vi "Open Selected VI Location.vi"(6 "Variant in":variant, 7 "Shift Pressed?":bool, 8 "error in (no error)":errorcluster, 10 "QD Combo Box Ref":refnum<vi>, 11 "QD Launch VI Ref":refnum<vi>) -> (0 "error out":errorcluster, 4 "Variant out":variant)   [LabVIEW 2017, in "Smart Open VI Location.lvlib"]
doc: "Open Selected VI's Location in Explorer Window."
uses:
  Smart Open VI Location.lvlib
panel:
  in  "Undo Name":string="Quick Drop Keyboard Shortcut"
  # "Do not change the connector pane of this VI.\n\nSee the block diagram for directions on how to use this template."
  # "Specify the name of the Undo transaction"
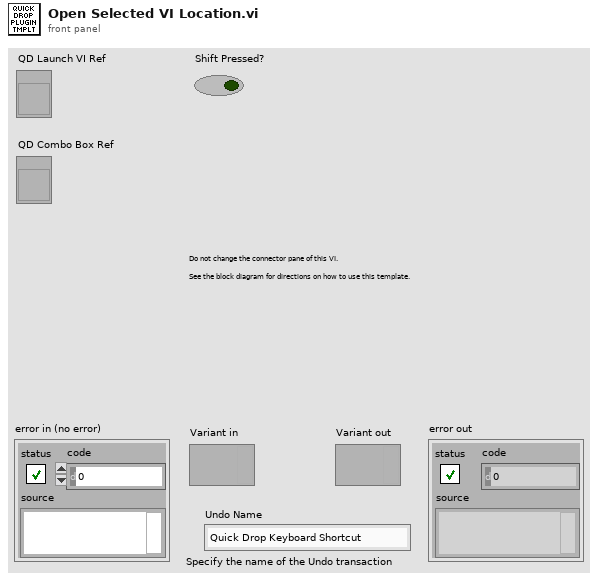
[diagram p1: front panel]
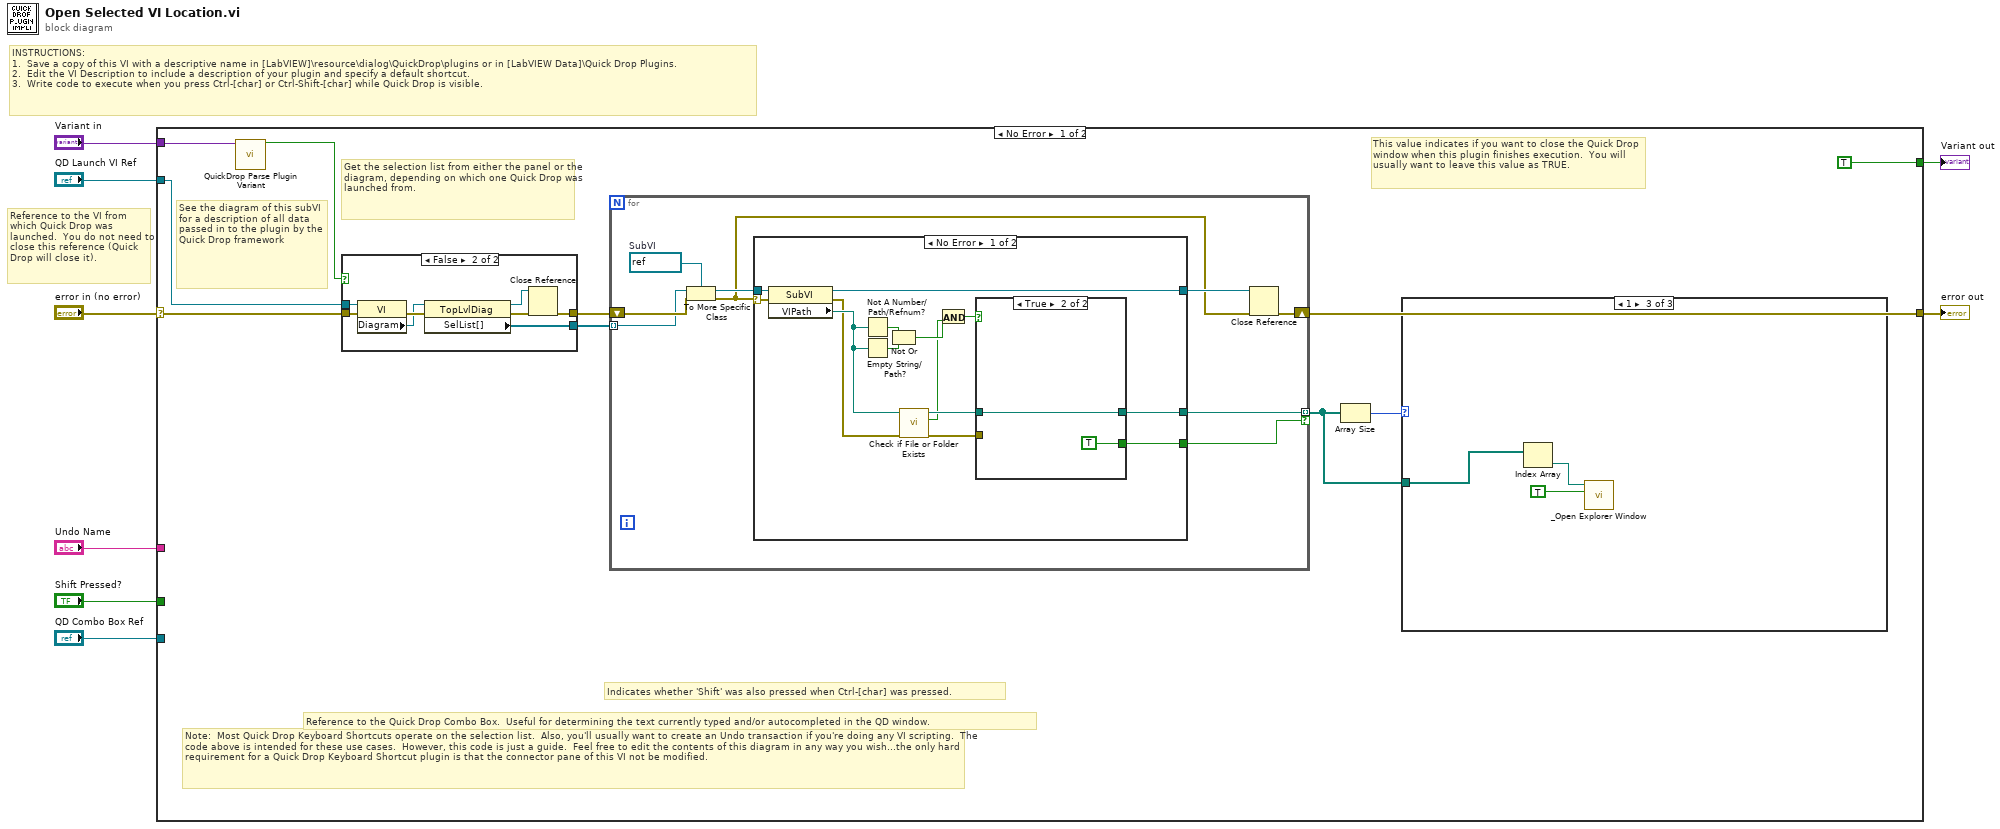
[diagram p0: block diagram]
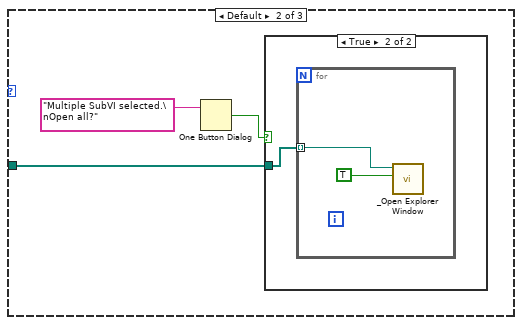
[diagram p3: hidden frame]
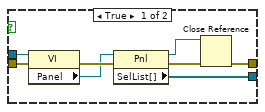
[diagram p7: hidden frame]
diagram:
  # "Reference to the VI from which Quick Drop was launched.  You do not need to close this reference (Quick Drop will close it)."
  # "INSTRUCTIONS:\n1.  Save a copy of this VI with a descriptive name in [LabVIEW]\\resource\\dialog\\QuickDrop\\plugins or in [LabVIEW Data]\\Quick Drop Plugins.\n2.  Edit the VI Description to include a description of your plugin and specify a default shortcut. \n3.  Write code to execute when you press Ctrl-[char] or Ctrl-Shift-[char] while Quick Drop is visible."
  n1 = case shown="No Error" "error in (no error)" {
    selector: "error in (no error)" -> [w17 w70]
    tunnel: [w11 w70] -> w7
    tunnel: "QD Launch VI Ref" -> [w16 _]
    tunnel: "Shift Pressed?" -> [_ _]
    tunnel: "QD Combo Box Ref" -> [_ _]
    tunnel: "Variant in" -> [w18 _]
    tunnel: "Undo Name" -> [_ _]
    tunnel: [TRUE _] -> w1
    frame No Error {
      # "Note:  Most Quick Drop Keyboard Shortcuts operate on the selection list.  Also, you'll usually want to create an Undo transaction if you're doing any VI scripting.  The code above is intended for these use cases.  However, this code is just a guide.  Feel free to edit the contents of this diagram in any way you wish...the only hard requirement for a Quick Drop Keyboard Shortcut plugin is that the connector pane of this VI not be modified."
      # "Get the selection list from either the panel or the diagram, depending on which one Quick Drop was launched from."
      # "This value indicates if you want to close the Quick Drop window when this plugin finishes execution.  You will usually want to leave this value as TRUE."
      # "See the diagram of this subVI for a description of all data passed in to the plugin by the Quick Drop framework"
      # "Reference to the Quick Drop Combo Box.  Useful for determining the text currently typed and/or autocompleted in the QD window."
      # "Indicates whether 'Shift' was also pressed when Ctrl-[char] was pressed."
      n2 = call <vilib>:"QuickDrop Parse Plugin Variant.vi"("QDKS Variant in"=w18) -> ("QD Launch VI Panel?"=w14:bool)  [unwired: 12 in, 2 out]
      n3 = case shown="False" w14 {
        tunnel: w17 -> [w61 w69]
        tunnel: w16 -> [w60 w68]
        tunnel: [w55 w63] -> w13
        tunnel: [w54 w62] -> w12
        frame True {
          n4 = property class="VI"(reference=w60, error in=w61) -> (error out=w59:errorcluster, "Panel"=w58:refnum<vi>)  [unwired: 1 out]
          n5 = property class="Pnl"(reference=w58, error in=w59) -> (reference out=w56:refnum<vi>, error out=w57:errorcluster, "SelList[]"=w54:refnum<vi>[])
          n6 = Close Reference(reference=w56, error in (no error)=w57) -> (error out=w55:errorcluster)
        }
        frame False {
          n7 = property class="VI"(reference=w68, error in=w69) -> (error out=w67:errorcluster, "Diagram"=w66:refnum<vi>)  [unwired: 1 out]
          n8 = property class="TopLvlDiag"(reference=w66, error in=w67) -> (reference out=w64:refnum<vi>, error out=w65:errorcluster, "SelList[]"=w62:refnum<vi>[])
          n9 = Close Reference(reference=w64, error in (no error)=w65) -> (error out=w63:errorcluster)
        }
      }
      n10 = for {
        shift-right: [w36] -> w11
        shift-left: w13 -> [w34]
        tunnel: w12 -> [w33] mode=indexing
        tunnel: [w29] -> w9 mode=indexing if=w28
        w30 = refnum<vi> refnum  # SubVI
        n11 = To More Specific Class(target class=w30, reference=w33, error in=w34) -> (specific class reference=w32:refnum<vi>, error out=w31:errorcluster)
        n12 = case shown="No Error" w31 {
          selector: w31 -> [w49 _]
          tunnel: [w50 w53] -> w35
          tunnel: w32 -> [w48 w53]
          tunnel: [w40 _] -> w29
          tunnel: [w39 _] -> w28
          frame No Error {
            n13 = property class="SubVI"(reference=w48, error in=w49) -> (reference out=w50:refnum<vi>, error out=w41:errorcluster, "VIPath"=w42:path)
            n14 = Not A Number/Path/Refnum?(number/path/refnum=w42) -> (NaN/Path/Refnum?=w38:bool)
            n15 = Empty String/Path?(string/path=w42) -> (empty?=w37:bool)
            n16 = Not Or(1:w37, 2:w38) -> (0:w45:bool)
            n17 = call <vilib>:"Check if File or Folder Exists.vi"("error in (no error)"=w41, "path"=w42) -> ("error out"=w46:errorcluster, "file or folder exists?"=w44:bool, "dup path"=w47:path)  [unwired: 7 in]
            n18 = And(x=w45, y=w44) -> (x .and. y?=w43:bool)
            n19 = case shown="True" w43 {
              tunnel: w47 -> [_ w52]
              tunnel: w46 -> [_ _]
              tunnel: [_ w52] -> w40
              tunnel: [_ TRUE] -> w39
              frame False {
              }
              frame True {
              }
            }
          }
          frame Error {
          }
        }
        n20 = Close Reference(reference=w35, error in (no error)=w31) -> (error out=w36:errorcluster)
      }
      n21 = Array Size(array=w9) -> (size(s)=w10:i32)
      n22 = case shown="1" w10 {
        tunnel: w9 -> [_ w20 w26]
        frame 0 {
        }
        frame Default {
          n23 = One Button Dialog(message="Multiple SubVI selected.\nOpen all?") -> (true=w19:bool)  [unwired: 1 in]
          n24 = case shown="True" w19 {
            tunnel: w20 -> [_ w22]
            frame False {
            }
            frame True {
              n25 = for {
                tunnel: w22 -> [w23] mode=indexing
                n26 = call "_Open Explorer Window.vi"("Select Directory? (F: Open Directory)"=TRUE, "Directory or File"=w23) -> ()  [unwired: 9 in, 1 out]
              }
            }
          }
        }
        frame 1 {
          n27 = Index Array(array=w26) -> (element=w25:path)  [unwired: 1 in]
          n28 = call "_Open Explorer Window.vi"("Select Directory? (F: Open Directory)"=TRUE, "Directory or File"=w25) -> ()  [unwired: 9 in, 1 out]
        }
      }
    }
    frame Error {
    }
  }
  "error out" <- w7
  "Variant out" <- w1
